vi "fgv_wfm_config.vi"(7 "cmd":T2, 11 "wfm config":T1={"history size"=60, "dim"=730, "StartCursor X"=0.0, "EndCursor X"=0.0, "ZeroCursor X"=0.0}) -> (3 "wfm config 2":T1={"history size"=60, "dim"=730, "StartCursor X"=0.0, "EndCursor X"=0.0, "ZeroCursor X"=0.0})   [LabVIEW 2021]
uses:
  ctrl/rw.ctl
  ctrl/wfm_cfg.ctl
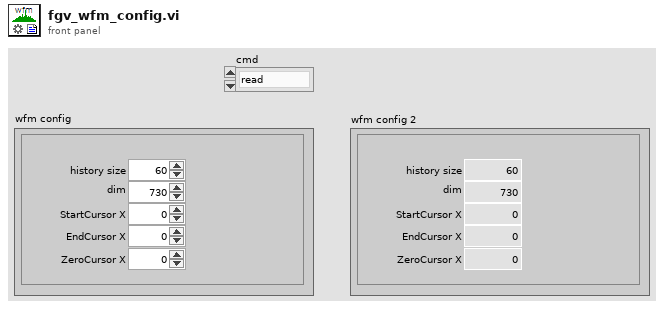
[diagram p1: front panel]
types:
  T1 = typedef "wfm_cfg.ctl" = cluster{"history size":i32, "dim":i32, "StartCursor X":dbl, "EndCursor X":dbl, "ZeroCursor X":dbl}
  T2 = typedef "rw.ctl" = enum16{"read", "write"}
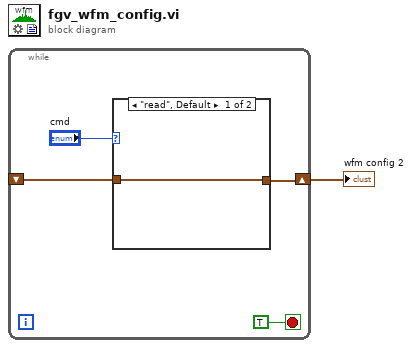
[diagram p0: block diagram]
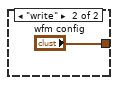
[diagram p2: hidden frame]
diagram:
  n1 = while {
    shift-right: [w3] -> w1
    shift-left: _ -> [w2]
    stop <- TRUE stop-if-true
    n2 = case shown="\"read\", Default" "cmd" {
      tunnel: [w6 "wfm config"] -> w3
      tunnel: w2 -> [w6 _]
      frame "read", Default {
      }
      frame "write" {
      }
    }
  }
  "wfm config 2" <- w1
